vi "Loop.vi"(9 "Error Queue":refnum<queue>, 10 "Helper Loop Queue":refnum<queue>, 11 "Helper Loop in":refnum<class "Event Actor.lvclass">) -> ()   [LabVIEW 2021, in "Event Actor.lvclass"]
uses:
  Event Actor.lvclass
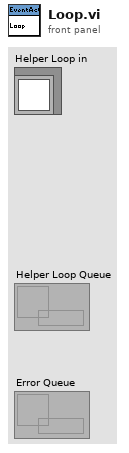
[diagram p1: front panel]
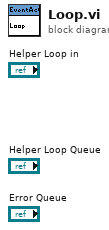
[diagram p0: block diagram]
diagram:
